vi "Response Parameters FG.vi"(7 "Action":T1, 8 "error in (no error)":errorcluster, 10 "Reponse Parameters":T3={"Response"="", "Linked Channels"=[], "Type Value"=1.0, "Wait Type"=enum."Wait sec", "Use Channel"=FALSE, "Channel Path"=""}, 11 "Item Ref in":T2 format="%.0x") -> (0 "error out":errorcluster={"status"=TRUE, "code"=1172, "source"="Invoke Node Error calling static method NationalInstruments.VeriStand.SystemDefinitionAPI.NodeIDUtil.IDToCustomDeviceBase, (System.Reflection.TargetInvocationException: Exception has been thrown by the target of an invocation.\n\tInner Exception: System.Exception: NI VeriStand Error: 36, The specified Item Ref is invalid. The Item Ref refers to an item that doesn't exist) <append><b>System.Exception</b> in Custom Device Offline API.lvlib:ID To Custom Device Base.vi->Custom Device Offline API.lvlib:Get Item Property (Variant).vi->Custom Device API.lvlib:Get Item Property (Variant).vi->Instrument Addon Shared.lvlib:Response Parameters FG.vi"}, 2 "Response Parameters":T3={"Response"="", "Linked Channels"=[], "Type Value"=1.0, "Wait Type"=enum."Wait sec", "Use Channel"=FALSE, "Channel Path"=""}, 3 "Item Ref out":T2 format="%.0x")   [LabVIEW 2018, in "Instrument Addon Shared.lvlib"]
uses:
  Instrument Addon Shared.lvlib
  Types/Response Parameters.ctl
  Types/Linked Channel Cluster.ctl
  Types/Response Wait Type.ctl
  <vilib>/NI Veristand/Custom Device API/Custom Device Item Ref.ctl
  Types/FG Control.ctl
  Constants.vi
  <vilib>/NI Veristand/Custom Device API/Get Item Property (String).vi
  <vilib>/NI Veristand/Custom Device API/Get Item Property (String Array).vi
  <vilib>/NI Veristand/Custom Device API/Get Item Property (Double).vi
  <vilib>/NI Veristand/Custom Device API/Get Item Property (U32).vi
  <vilib>/NI Veristand/Custom Device API/Get Item Property (Boolean).vi
  <vilib>/NI Veristand/Custom Device API/Set Item Property (String).vi
  <vilib>/NI Veristand/Custom Device API/Set Item Property (String Array).vi
  <vilib>/NI Veristand/Custom Device API/Set Item Property (Double).vi
  <vilib>/NI Veristand/Custom Device API/Set Item Property (U32).vi
  <vilib>/NI Veristand/Custom Device API/Set Item Property (Boolean).vi
  <vilib>/NI Veristand/Custom Device API/Custom Device API.lvlib
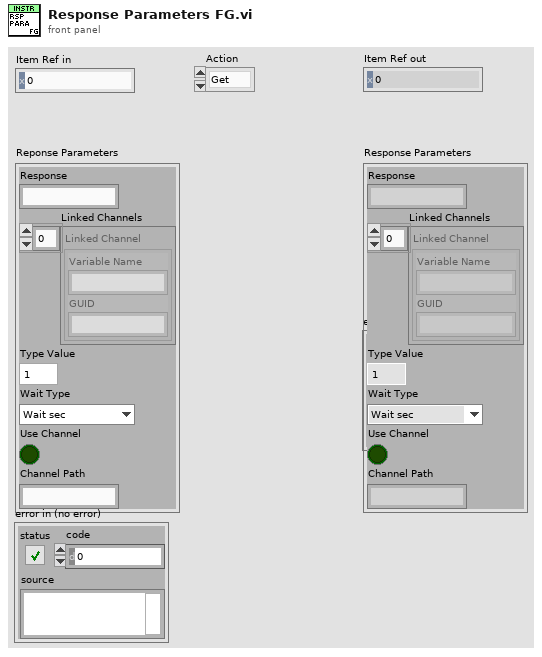
[diagram p1: front panel]
types:
  T1 = typedef "Instrument Addon Shared.lvlib/FG Control.ctl" = enum16{"Get", "Set"}
  T2 = typedef "Custom Device API.lvlib/Custom Device Item Ref.ctl" = u64
  T3 = typedef "Instrument Addon Shared.lvlib/Response Parameters.ctl" = cluster{"Response":string, "Linked Channels":T4[], "Type Value":dbl, "Wait Type":T5, "Use Channel":bool, "Channel Path":string}
  T4 = typedef "Instrument Addon Shared.lvlib/Linked Channel Cluster.ctl" = cluster{"Variable Name":string, "GUID":string}
  T5 = typedef "Instrument Addon Shared.lvlib/Response Wait Type.ctl" = enum16{"Byte Count", "Wait sec"}
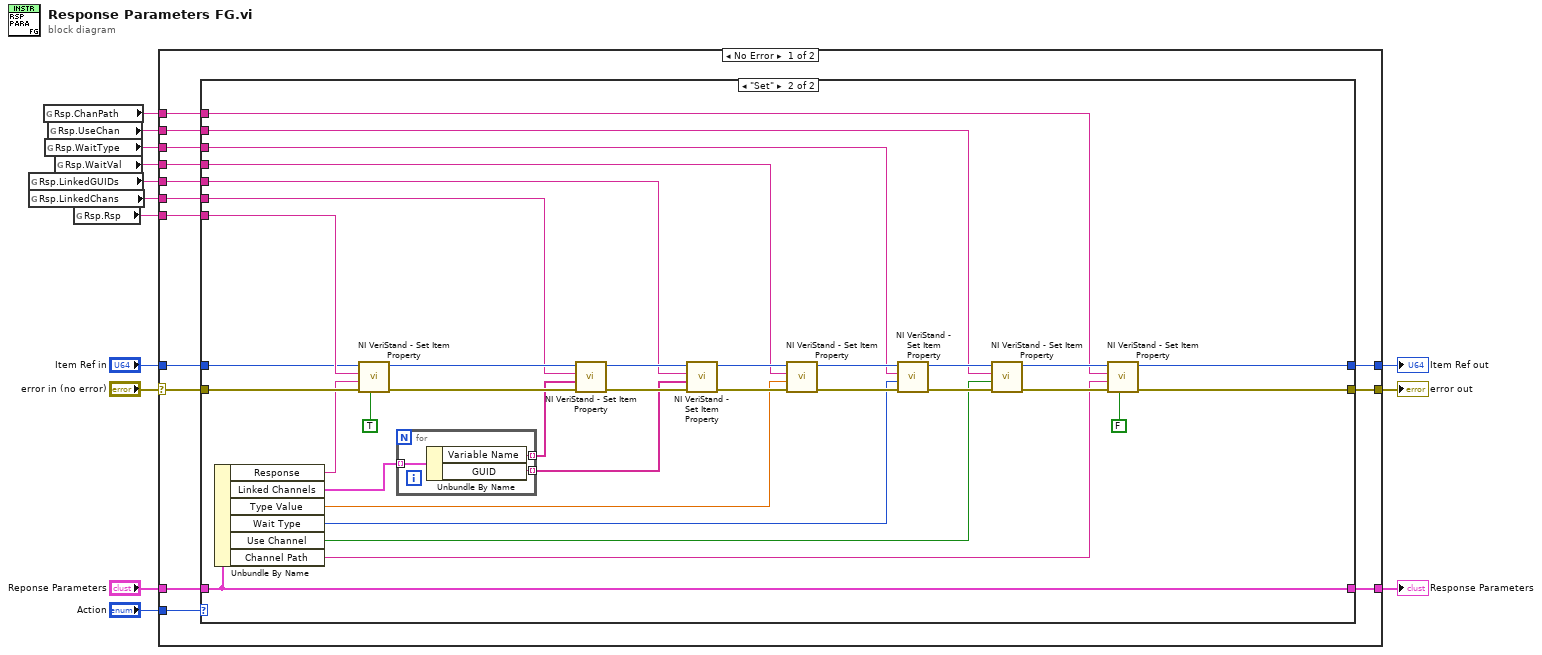
[diagram p0: block diagram]
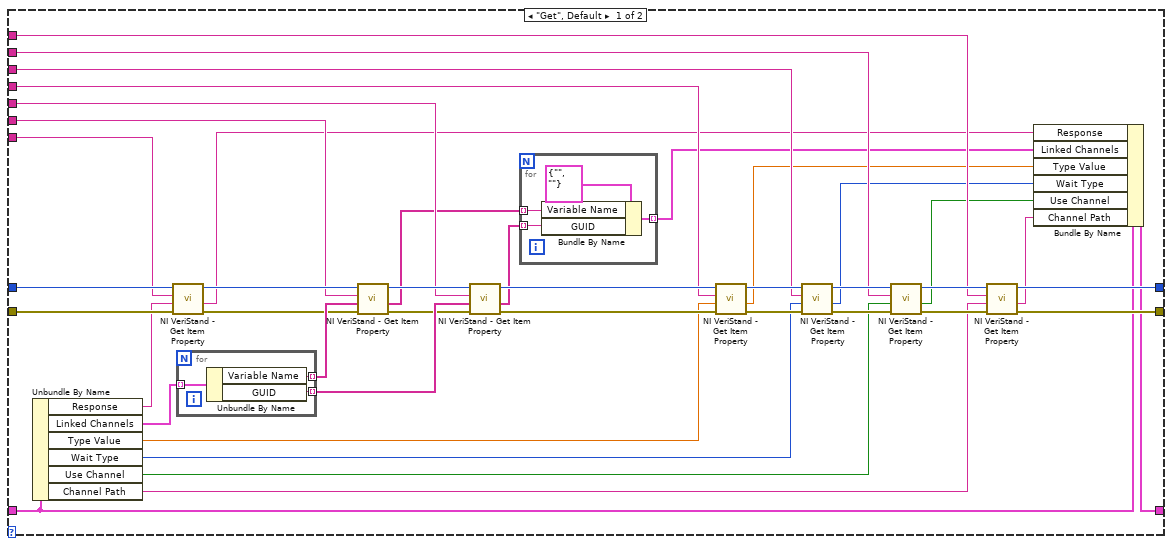
[diagram p2: hidden frame]
diagram:
  n1 = global read "Constants.vi" "Rsp.LinkedGUIDs"() -> (w5:string)
  n2 = global read "Constants.vi" "Rsp.LinkedChans"() -> (w6:string)
  n3 = global read "Constants.vi" "Rsp.ChanPath"() -> (w1:string)
  n4 = global read "Constants.vi" "Rsp.WaitType"() -> (w3:string)
  n5 = global read "Constants.vi" "Rsp.UseChan"() -> (w2:string)
  n6 = global read "Constants.vi" "Rsp.WaitVal"() -> (w4:string)
  n7 = global read "Constants.vi" "Rsp.Rsp"() -> (w8:string)
  n8 = case shown="No Error" "error in (no error)" {
    selector: "error in (no error)" -> [w23 w116]
    tunnel: w8 -> [w28 _]
    tunnel: [w27 w114] -> w12
    tunnel: "Item Ref in" -> [w26 w114]
    tunnel: "Reponse Parameters" -> [w25 w115]
    tunnel: [w24 w116] -> w11
    tunnel: [w22 w115] -> w7
    tunnel: "Action" -> [w21 _]
    tunnel: w6 -> [w20 _]
    tunnel: w5 -> [w19 _]
    tunnel: w4 -> [w18 _]
    tunnel: w3 -> [w17 _]
    tunnel: w2 -> [w16 _]
    tunnel: w1 -> [w15 _]
    frame No Error {
      n9 = case shown="\"Set\"" w21 {
        tunnel: w28 -> [w67 w110]
        tunnel: [w37 w98] -> w27
        tunnel: w26 -> [w68 w109]
        tunnel: w25 -> [w36 w107]
        tunnel: [w38 w99] -> w24
        tunnel: w23 -> [w69 w108]
        tunnel: [w35 w107] -> w22
        tunnel: w20 -> [w51 w87]
        tunnel: w19 -> [w49 w86]
        tunnel: w18 -> [w45 w84]
        tunnel: w17 -> [w44 w83]
        tunnel: w16 -> [w42 w81]
        tunnel: w15 -> [w39 w78]
        frame "Get", Default {
          n10 = Unbundle By Name(w36) -> ("Response"=w66:string, "Linked Channels"=w65:T4[], "Type Value"=w46:dbl, "Wait Type"=w43:T5, "Use Channel"=w41:bool, "Channel Path"=w40:string)
          n11 = call-poly <vilib>:"NI VeriStand - Get Item Property.vi"("error in (no error)"=w69, "Default Value"=w66, "Property Name"=w67, "Item Ref in"=w68) -> ("error out"=w57:errorcluster, "Value"=w34:string, "Item Ref out"=w62:T2)  [unwired: 4 in, 1 out]
          n12 = for {
            tunnel: w65 -> [w76] mode=indexing
            tunnel: [w75] -> w64 mode=indexing
            tunnel: [w74] -> w63 mode=indexing
            n13 = Unbundle By Name(w76) -> ("Variable Name"=w75:string, "GUID"=w74:string)
          }
          n14 = call-poly <vilib>:"NI VeriStand - Get Item Property.vi"("error in (no error)"=w57, "Default Value"=w64, "Property Name"=w51, "Item Ref in"=w62) -> ("error out"=w56:errorcluster, "Value"=w48:string[], "Item Ref out"=w50:T2)  [unwired: 4 in, 1 out]
          n15 = call-poly <vilib>:"NI VeriStand - Get Item Property.vi"("error in (no error)"=w56, "Default Value"=w63, "Property Name"=w49, "Item Ref in"=w50) -> ("error out"=w55:errorcluster, "Value"=w47:string[], "Item Ref out"=w61:T2)  [unwired: 4 in, 1 out]
          n16 = for {
            tunnel: w47 -> [w71] mode=indexing
            tunnel: w48 -> [w70] mode=indexing
            tunnel: [w72] -> w33 mode=indexing
            n17 = Bundle By Name(cluster=T4 {"Variable Name"="", "GUID"=""} ("Linked Channel"), "Variable Name"=w70, "GUID"=w71) -> (w72:T4)
          }
          n18 = call-poly <vilib>:"NI VeriStand - Get Item Property.vi"("error in (no error)"=w55, "Default Value"=w46, "Property Name"=w45, "Item Ref in"=w61) -> ("error out"=w54:errorcluster, "Value"=w32:dbl, "Item Ref out"=w60:T2)  [unwired: 4 in, 1 out]
          n19 = call-poly <vilib>:"NI VeriStand - Get Item Property.vi"("error in (no error)"=w54, "Default Value"=w43, "Property Name"=w44, "Item Ref in"=w60) -> ("error out"=w53:errorcluster, "Value"=w31:u32, "Item Ref out"=w59:T2)  [unwired: 4 in, 1 out]
          n20 = call-poly <vilib>:"NI VeriStand - Get Item Property.vi"("error in (no error)"=w53, "Default Value"=w41, "Property Name"=w42, "Item Ref in"=w59) -> ("error out"=w52:errorcluster, "Value"=w30:bool, "Item Ref out"=w58:T2)  [unwired: 4 in, 1 out]
          n21 = call-poly <vilib>:"NI VeriStand - Get Item Property.vi"("error in (no error)"=w52, "Default Value"=w40, "Property Name"=w39, "Item Ref in"=w58) -> ("error out"=w38:errorcluster, "Value"=w29:string, "Item Ref out"=w37:T2)  [unwired: 4 in, 1 out]
          n22 = Bundle By Name(cluster=w36, "Response"=w34, "Linked Channels"=w33, "Type Value"=w32, "Wait Type"=w31, "Use Channel"=w30, "Channel Path"=w29) -> (w35:T3)
        }
        frame "Set" {
          n23 = Unbundle By Name(w107) -> ("Response"=w106:string, "Linked Channels"=w90:T4[], "Type Value"=w85:dbl, "Wait Type"=w82:T5, "Use Channel"=w80:bool, "Channel Path"=w79:string)
          n24 = call-poly <vilib>:"NI VeriStand - Set Item Property.vi"("Binary String (T)"=TRUE, "error in (no error)"=w108, "Value"=w106, "Property Name"=w110, "Item Ref in"=w109) -> ("error out"=w100:errorcluster, "Item Ref out"=w97:T2)  [unwired: 4 in, 1 out]
          n25 = for {
            tunnel: w90 -> [w113] mode=indexing
            tunnel: [w112] -> w89 mode=indexing
            tunnel: [w111] -> w88 mode=indexing
            n26 = Unbundle By Name(w113) -> ("Variable Name"=w112:string, "GUID"=w111:string)
          }
          n27 = call-poly <vilib>:"NI VeriStand - Set Item Property.vi"("error in (no error)"=w100, "Value"=w89, "Property Name"=w87, "Item Ref in"=w97) -> ("error out"=w105:errorcluster, "Item Ref out"=w96:T2)  [unwired: 5 in, 1 out]
          n28 = call-poly <vilib>:"NI VeriStand - Set Item Property.vi"("error in (no error)"=w105, "Value"=w88, "Property Name"=w86, "Item Ref in"=w96) -> ("error out"=w104:errorcluster, "Item Ref out"=w95:T2)  [unwired: 5 in, 1 out]
          n29 = call-poly <vilib>:"NI VeriStand - Set Item Property.vi"("error in (no error)"=w104, "Value"=w85, "Property Name"=w84, "Item Ref in"=w95) -> ("error out"=w103:errorcluster, "Item Ref out"=w94:T2)  [unwired: 5 in, 1 out]
          n30 = call-poly <vilib>:"NI VeriStand - Set Item Property.vi"("error in (no error)"=w103, "Value"=w82, "Property Name"=w83, "Item Ref in"=w94) -> ("error out"=w102:errorcluster, "Item Ref out"=w93:T2)  [unwired: 5 in, 1 out]
          n31 = call-poly <vilib>:"NI VeriStand - Set Item Property.vi"("error in (no error)"=w102, "Value"=w80, "Property Name"=w81, "Item Ref in"=w93) -> ("error out"=w101:errorcluster, "Item Ref out"=w92:T2)  [unwired: 5 in, 1 out]
          n32 = call-poly <vilib>:"NI VeriStand - Set Item Property.vi"("Binary String (T)"=FALSE, "error in (no error)"=w101, "Value"=w79, "Property Name"=w78, "Item Ref in"=w92) -> ("error out"=w99:errorcluster, "Item Ref out"=w98:T2)  [unwired: 4 in, 1 out]
        }
      }
    }
    frame Error {
    }
  }
  "error out" <- w11
  "Response Parameters" <- w7
  "Item Ref out" <- w12
